vi "digital2string.vi"(10 "数值":u32 format="%x") -> (2 "字符串":string)   [LabVIEW 2017]
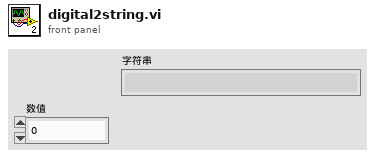
[diagram p1: front panel]
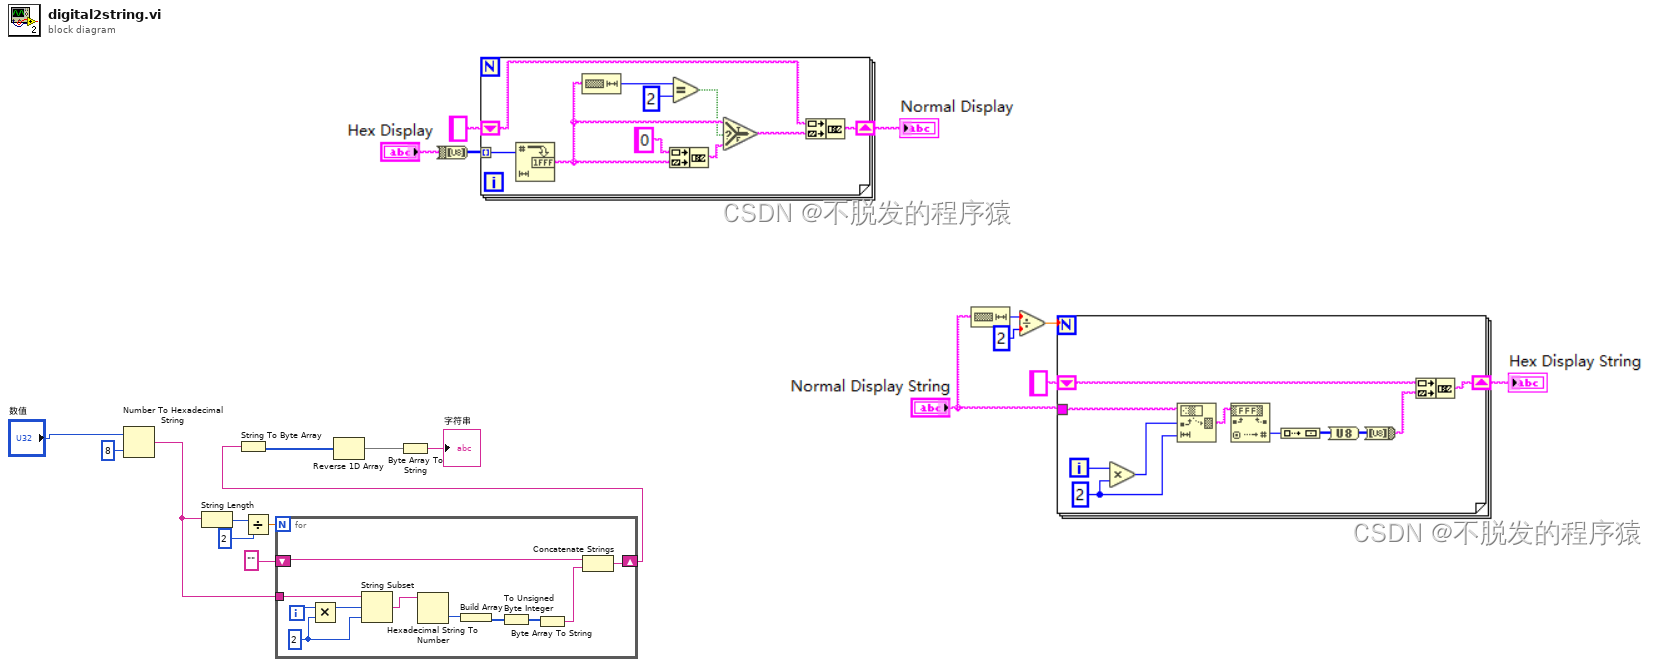
[diagram p0: block diagram]
diagram:
  n1 = Number To Hexadecimal String(1:i16 8 ("宽度(-)"), 2:"数值") -> (0:w2:string)
  n2 = String Length(string=w2) -> (length=w5:i32)
  n3 = Divide(x=w5, y=2) -> (x/y=w6:dbl)
  n4 = for {
    N: w6 -> [_]
    shift-right: [w14] -> w1
    shift-left: "" -> [w12]
    tunnel: w2 -> [w22]
    i -> [w21]
    w19 = 2 ("y")
    n5 = Multiply(x=w21, y=w19) -> (x*y=w20:i32)
    n6 = String Subset(string=w22, offset (0)=w20, length (rest)=w19) -> (substring=w18:string)
    n7 = Hexadecimal String To Number(string=w18) -> (number=w17:u32)  [unwired: 2 in, 1 out]
    n8 = Build Array(w17) -> (w16:u32[])
    n9 = To Unsigned Byte Integer(number=w16) -> (unsigned 8bit integer=w15:u8[])
    n10 = Byte Array To String(unsigned byte array=w15) -> (string=w13:string)
    n11 = Concatenate Strings(w12, w13) -> (w14:string)
  }
  n12 = String To Byte Array(string=w1) -> (unsigned byte array=w9:u8[])
  n13 = Reverse 1D Array(array=w9) -> (reversed array=w8:u8[])
  n14 = Byte Array To String(unsigned byte array=w8) -> (string=→"字符串":string)
